vi "CloseThisConnection.vi"(8 "error in (no error)":errorcluster, 11 "TCP_Client_Window in":refnum<class "TCP_Client_Window.lvclass">) -> (0 "error out":errorcluster, 3 "TCP_Client_Window out":refnum<class "TCP_Client_Window.lvclass">)   [LabVIEW 2023, in "TCP_Client_Window.lvlib" / "TCP_Client_Window.lvclass"]
uses:
  TCP_Client_Window.lvclass
  TCP_Client_Window.lvclass/TCP_Client_Window.ctl
  <vilib>/ActorFramework/Actor/Actor.lvclass
  TCP_ClientWindow_Controller Messages/CloseConnection Msg/CloseConnection Msg.lvclass
  C:/Program Files (x86)/National Instruments/LabVIEW 2023/vi.lib/ActorFramework/Actor/Actor.lvclass
  C:/Source/LabVIEW/TCP_server/TCP_Client_Window/TCP_Client_Window/TCP_Client_Window.lvclass
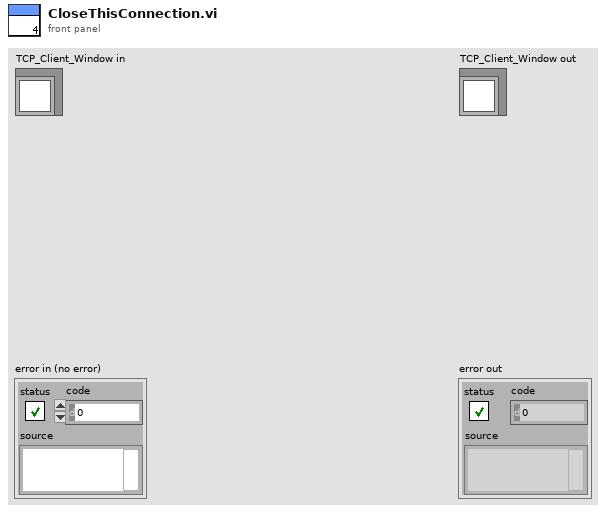
[diagram p1: front panel]
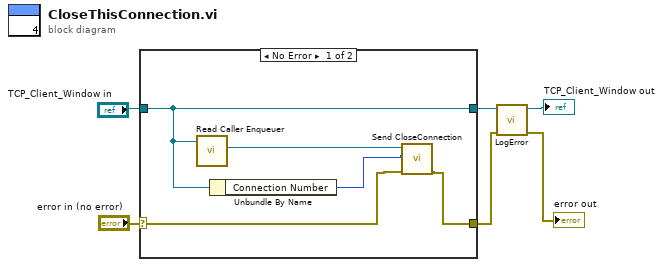
[diagram p0: block diagram]
diagram:
  n1 = case shown="No Error" "error in (no error)" {
    selector: "error in (no error)" -> [w8 w13]
    tunnel: [w7 w13] -> w3
    tunnel: [w11 w12] -> w4
    tunnel: "TCP_Client_Window in" -> [w11 w12]
    frame No Error {
      n2 = call <vilib>:"Read Caller Enqueuer.vi"("Actor"=w11) -> ("Caller Enqueuer"=w10:refnum<class "Message Enqueuer.lvclass">)  [unwired: 10 in]
      n3 = Unbundle By Name(w11) -> ("Connection Number"=w9:i32)
      n4 = call "Send CloseConnection.vi"("error in (no error)"=w8, "Connection number"=w9, "Message Enqueuer"=w10) -> ("error out"=w7:errorcluster)  [unwired: 7 in, 1 out]
    }
    frame Error {
    }
  }
  n5 = call "LogError.vi"("error in (no error)"=w3, "TCP_Client_Window in"=w4) -> ("error out"=→"error out":errorcluster, "TCP_Client_Window out"=→"TCP_Client_Window out":refnum<class "TCP_Client_Window.lvclass">)  [unwired: 8 in]
